vi "RemoteLoader.vi"() -> ()   [LabVIEW 2012]
uses:
  RemoteControl_class/RemoteControl.lvclass
  Light_class/Light.lvclass
  GarageDoor_class/GarageDoor.lvclass
  CeilingFan_class/CeilingFan.lvclass
  Command_class/Command.lvclass
  LightOnCommand_class/LightOnCommand.lvclass
  LightOffCommand_class/LightOffCommand.lvclass
  GarageDoorCloseCommand_class/GarageDoorCloseCommand.lvclass
  GarageDoorOpenCommand_class/GarageDoorOpenCommand.lvclass
  CeilingFanHighCommand_class/CeilingFanHighCommand.lvclass
  CeilingFanLowCommand_class/CeilingFanLowCommand.lvclass
  <userlib>/_LabVIEWCommon/LcError/LcAbort/LcAbort.lvclass
panel:
  in  "stop":bool
  out "error out":errorcluster
  in  "error in (no error)":errorcluster
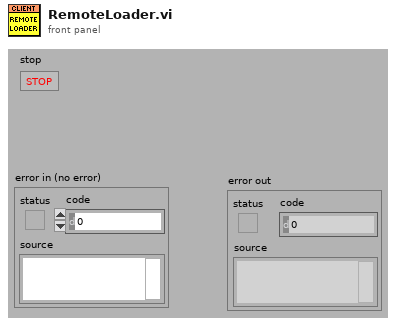
[diagram p1: front panel]
types:
  T1 = cluster{"Remote":refnum<class "RemoteControl.lvclass">, "Light":refnum<class "Light.lvclass">, "GarageDoor":refnum<class "GarageDoor.lvclass">, "CeilingFan":refnum<class "CeilingFan.lvclass">}
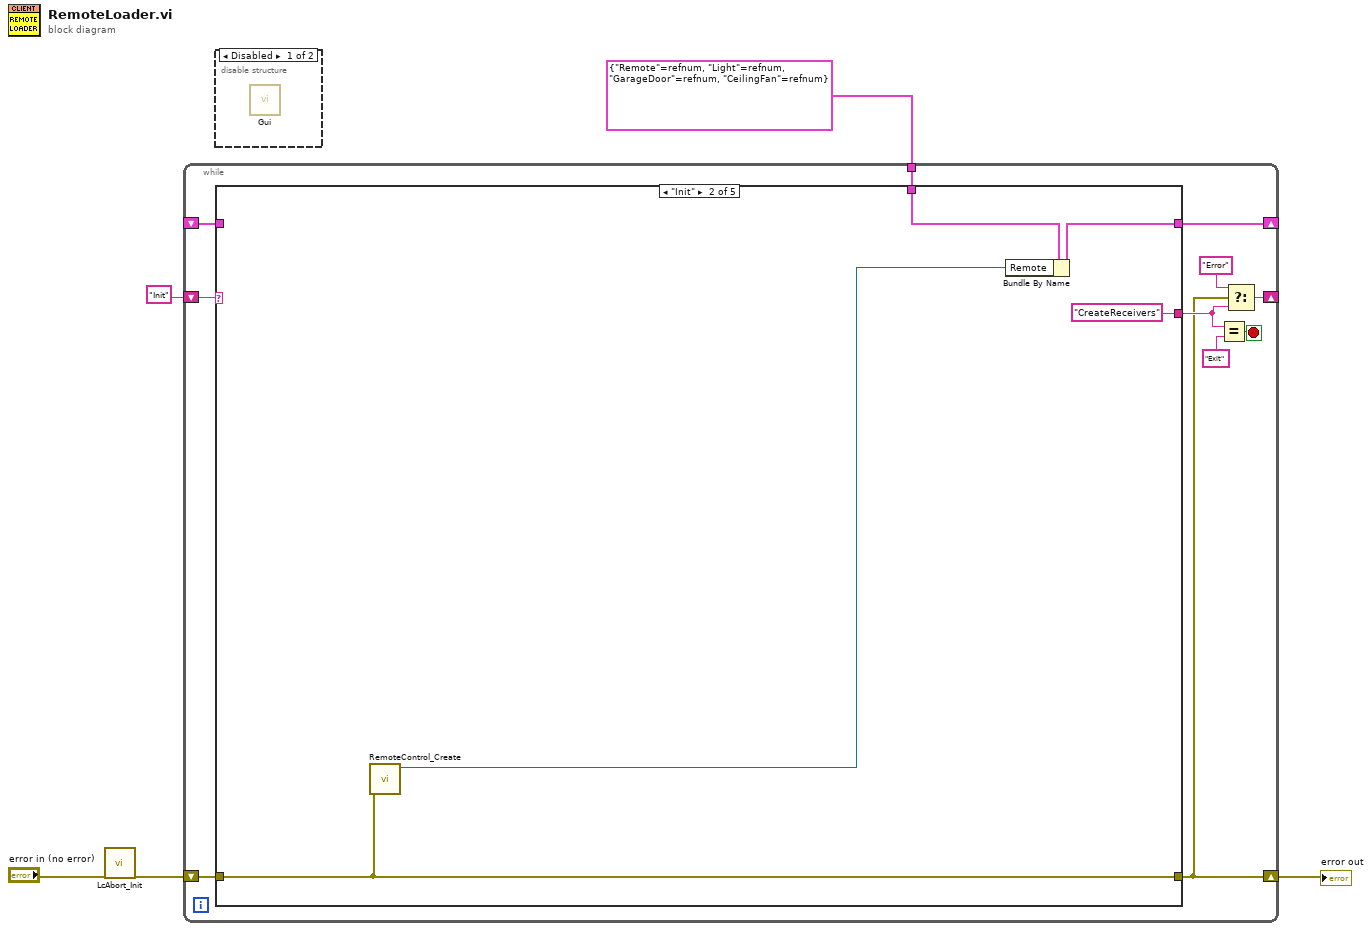
[diagram p0: block diagram]
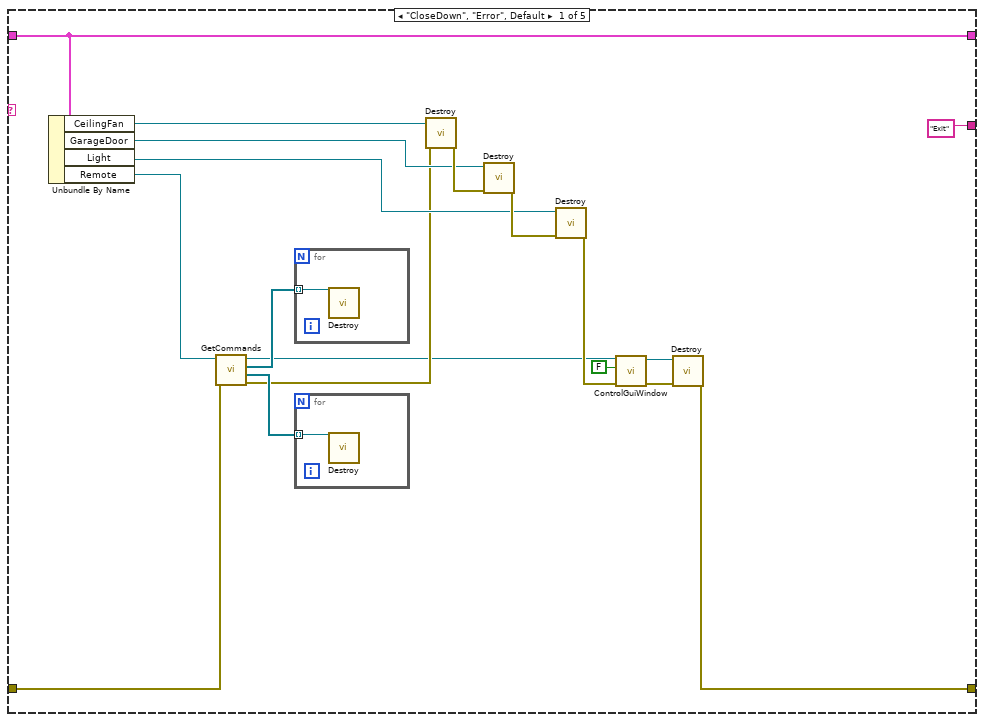
[diagram p3: hidden frame]
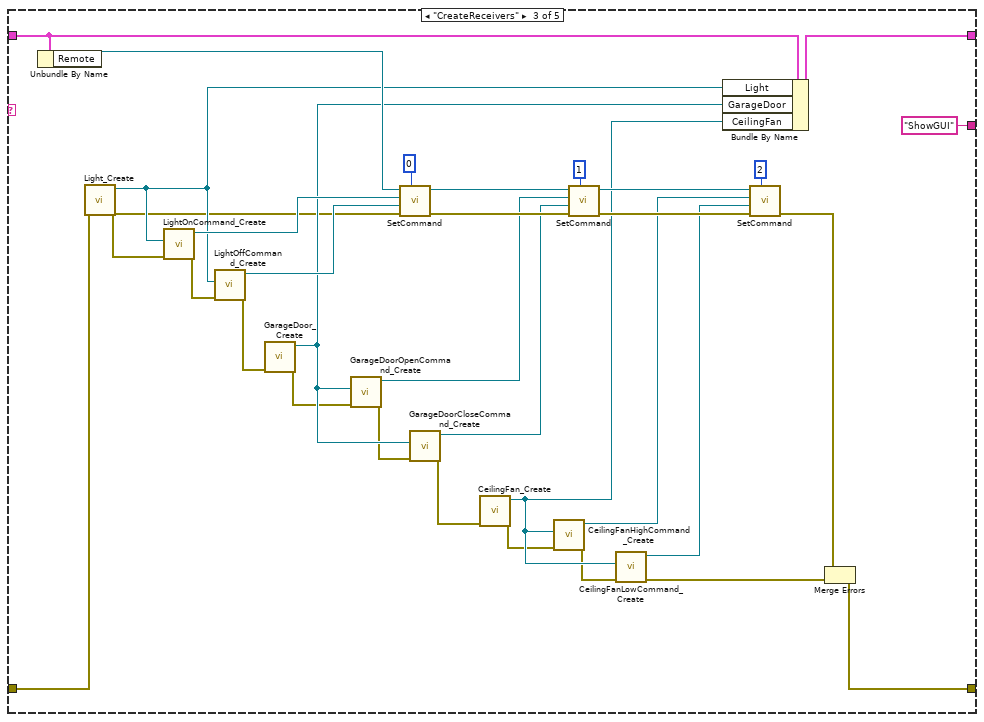
[diagram p4: hidden frame]
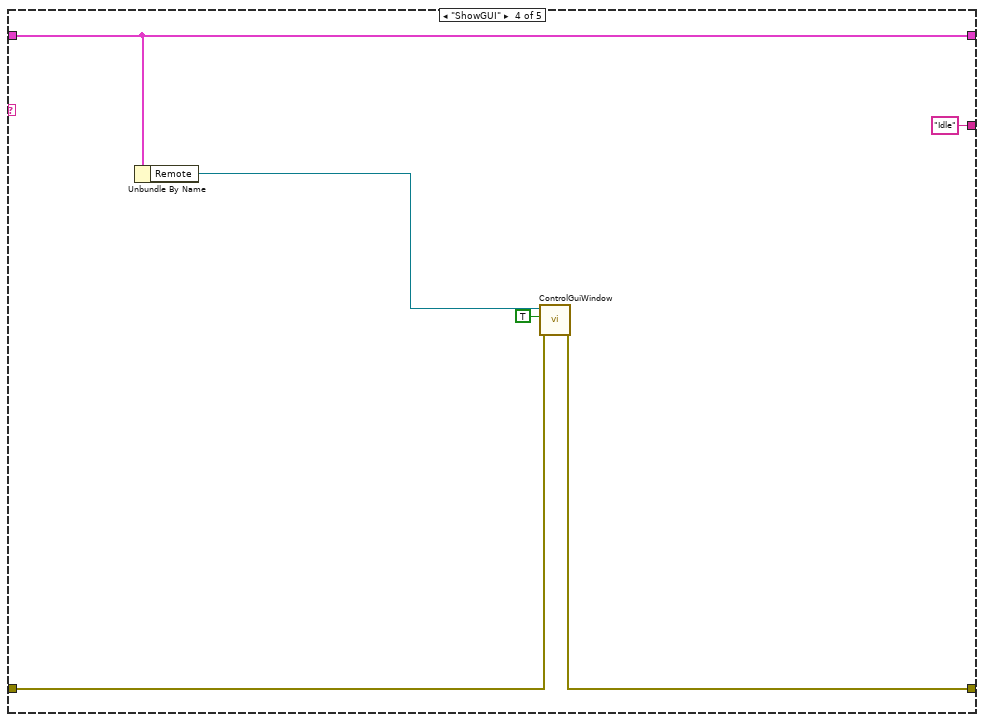
[diagram p5: hidden frame]
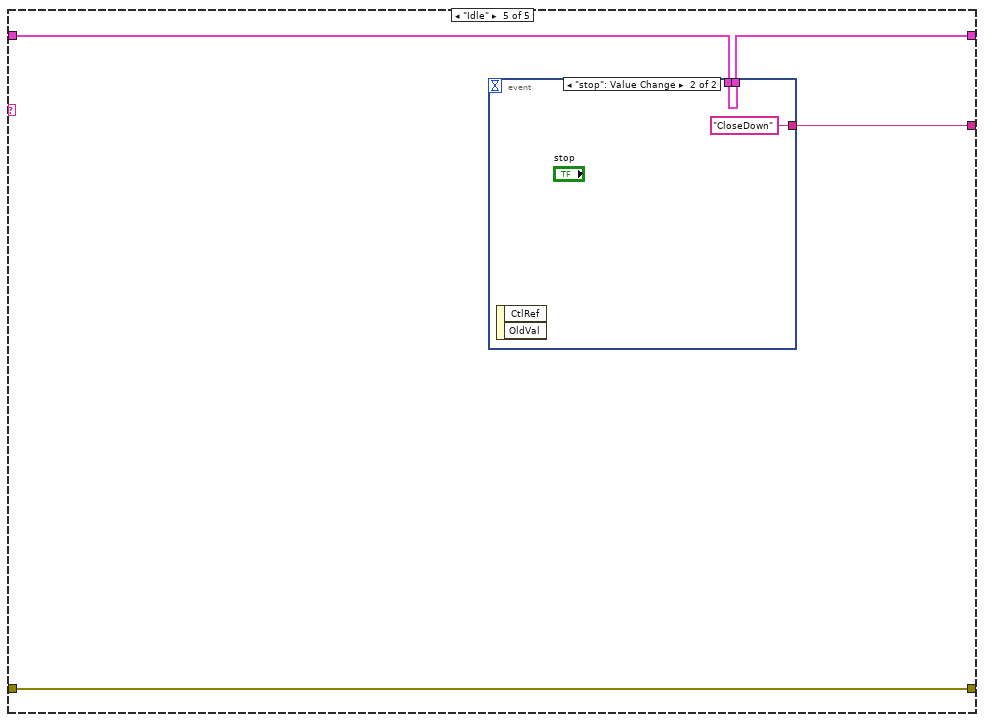
[diagram p6: hidden frame]
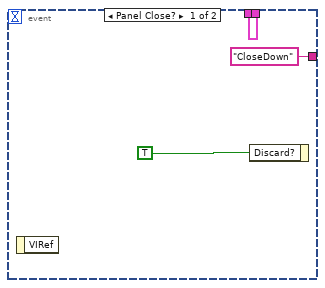
[diagram p7: hidden frame]
diagram:
  n1 = call <userlib>:"LcAbort_Init.vi"("error in (no error)"="error in (no error)") -> ("error out"=w1:errorcluster)  [unwired: 18 in]
  n2 = while {
    shift-right: [w9] -> w4
    shift-left: w1 -> [w16]
    shift-right: [w14] -> _
    shift-left: "Init" -> [w15]
    shift-right: [w8] -> _
    shift-left: _ -> [w7]
    tunnel: T1 {"Remote"=refnum, "Light"=refnum, "GarageDoor"=refnum, "CeilingFan"=refnum} -> [w6]
    stop <- w13 stop-if-true
    n3 = case shown="\"Init\"" w15 {
      tunnel: w16 -> [w19 w39 w57 w79 w80]
      tunnel: [w18 w39 w49 w76 w80] -> w9
      tunnel: ["Exit" "CreateReceivers" "ShowGUI" "Idle" w81] -> w10
      tunnel: [w33 w40 w47 w74 w82] -> w8
      tunnel: w7 -> [w33 _ w48 w74 w83]
      tunnel: w6 -> [_ w37 _ _ _]
      frame "CloseDown", "Error", Default {
        n4 = Unbundle By Name(w33) -> ("CeilingFan"=w32:refnum<class "CeilingFan.lvclass">, "GarageDoor"=w30:refnum<class "GarageDoor.lvclass">, "Light"=w28:refnum<class "Light.lvclass">, "Remote"=w17:refnum<class "RemoteControl.lvclass">)
        n5 = call-dynamic "GetCommands.vi"("error in (no error)"=w19, "reference in"=w17) -> ("error out"=w22:errorcluster, "OfCommands"=w23:refnum<class "Command.lvclass">[], "OnCommands"=w24:refnum<class "Command.lvclass">[], "reference out"=w21:refnum<class "RemoteControl.lvclass">)  [unwired: 6 in]
        n6 = for {
          tunnel: w24 -> [w36] mode=indexing
          n7 = call-dynamic "Destroy.vi"("reference in"=w36) -> ()  [unwired: 9 in, 2 out]
        }
        n8 = for {
          tunnel: w23 -> [w35] mode=indexing
          n9 = call-dynamic "Destroy.vi"("reference in"=w35) -> ()  [unwired: 9 in, 2 out]
        }
        n10 = call-dynamic "Destroy.vi"("error in (no error)"=w22, "reference in"=w32) -> ("error out"=w31:errorcluster)  [unwired: 8 in, 1 out]
        n11 = call-dynamic "Destroy.vi"("error in (no error)"=w31, "reference in"=w30) -> ("error out"=w29:errorcluster)  [unwired: 8 in, 1 out]
        n12 = call-dynamic "Destroy.vi"("error in (no error)"=w29, "reference in"=w28) -> ("error out"=w25:errorcluster)  [unwired: 8 in, 1 out]
        n13 = call "ControlGuiWindow.vi"("error in (no error)"=w25, "ShowProcessWindow"=FALSE, "reference in"=w21) -> ("error out"=w26:errorcluster, "reference out"=w27:refnum<class "RemoteControl.lvclass">)  [unwired: 7 in]
        n14 = call-dynamic "Destroy.vi"("error in (no error)"=w26, "reference in"=w27) -> ("error out"=w18:errorcluster)  [unwired: 8 in, 1 out]
      }
      frame "Init" {
        n15 = call "RemoteControl_Create.vi"("error in (no error)"=w39) -> ("reference out"=w38:refnum<class "RemoteControl.lvclass">)  [unwired: 9 in, 1 out]
        n16 = Bundle By Name(cluster=w37, "Remote"=w38) -> (w40:T1)
      }
      frame "CreateReceivers" {
        n17 = Unbundle By Name(w48) -> ("Remote"=w64:refnum<class "RemoteControl.lvclass">)
        n18 = call "Light_Create.vi"("error in (no error)"=w57) -> ("error out"=w52:errorcluster, "reference out"=w60:refnum<class "Light.lvclass">)  [unwired: 9 in]
        n19 = call "LightOnCommand_Create.vi"("error in (no error)"=w52, "Light"=w60) -> ("error out"=w72:errorcluster, "reference out"=w70:refnum<class "LightOnCommand.lvclass">)  [unwired: 8 in]
        n20 = call "LightOffCommand_Create.vi"("error in (no error)"=w72, "Light"=w60) -> ("error out"=w68:errorcluster, "reference out"=w69:refnum<class "LightOffCommand.lvclass">)  [unwired: 8 in]
        n21 = call "GarageDoor_Create.vi"("error in (no error)"=w68) -> ("error out"=w46:errorcluster, "reference out"=w59:refnum<class "GarageDoor.lvclass">)  [unwired: 9 in]
        n22 = call "GarageDoorOpenCommand_Create.vi"("error in (no error)"=w46, "GarageDoor"=w59) -> ("error out"=w45:errorcluster, "reference out"=w43:refnum<class "GarageDoorOpenCommand.lvclass">)  [unwired: 8 in]
        n23 = call-dynamic "SetCommand.vi"("ButtonIndex(0..n)"=0, "error in (no error)"=w52, "OffCommand"=w69, "OnCommand"=w70, "reference in"=w64) -> ("error out"=w65:errorcluster, "reference out"=w63:refnum<class "RemoteControl.lvclass">)  [unwired: 5 in]
        n24 = call "GarageDoorCloseCommand_Create.vi"("error in (no error)"=w45, "GarageDoor"=w59) -> ("error out"=w44:errorcluster, "reference out"=w42:refnum<class "GarageDoorCloseCommand.lvclass">)  [unwired: 8 in]
        n25 = call "CeilingFan_Create.vi"("error in (no error)"=w44) -> ("error out"=w56:errorcluster, "reference out"=w58:refnum<class "CeilingFan.lvclass">)  [unwired: 9 in]
        n26 = call "CeilingFanHighCommand_Create.vi"("error in (no error)"=w56, "CeilingFan"=w58) -> ("error out"=w55:errorcluster, "reference out"=w54:refnum<class "CeilingFanHighCommand.lvclass">)  [unwired: 8 in]
        n27 = call-dynamic "SetCommand.vi"("ButtonIndex(0..n)"=1, "error in (no error)"=w65, "OffCommand"=w42, "OnCommand"=w43, "reference in"=w63) -> ("error out"=w61:errorcluster, "reference out"=w62:refnum<class "RemoteControl.lvclass">)  [unwired: 5 in]
        n28 = call "CeilingFanLowCommand_Create.vi"("error in (no error)"=w55, "CeilingFan"=w58) -> ("error out"=w51:errorcluster, "reference out"=w53:refnum<class "CeilingFanLowCommand.lvclass">)  [unwired: 8 in]
        n29 = Bundle By Name(cluster=w48, "Light"=w60, "GarageDoor"=w59, "CeilingFan"=w58) -> (w47:T1)
        n30 = call-dynamic "SetCommand.vi"("ButtonIndex(0..n)"=2, "error in (no error)"=w61, "OffCommand"=w53, "OnCommand"=w54, "reference in"=w62) -> ("error out"=w50:errorcluster)  [unwired: 5 in, 1 out]
        n31 = Merge Errors(w50, w51) -> (w49:errorcluster)
      }
      frame "ShowGUI" {
        n32 = Unbundle By Name(w74) -> ("Remote"=w78:refnum<class "RemoteControl.lvclass">)
        n33 = call "ControlGuiWindow.vi"("error in (no error)"=w79, "ShowProcessWindow"=TRUE, "reference in"=w78) -> ("error out"=w76:errorcluster)  [unwired: 7 in, 1 out]
      }
      frame "Idle" {
        n34 = event shown="[1] \"stop\": Value Change" {
          selector: _ -> [_ _]
          dyn-events: _ -> [_ _]
          timeout: _ -> [_ _]
          tunnel: w83 -> [w84 w87]
          tunnel: [w84 w87] -> w82
          tunnel: ["CloseDown" "CloseDown"] -> w81
          event Panel Close? {
            n35 = event-data() -> ()  [unwired: 1 in, 1 out]
            n36 = event-data("Discard?"=TRUE) -> ()  [unwired: 1 in, 1 out]
          }
          event "stop": Value Change {
            n37 = event-data() -> ()  [unwired: 1 in, 2 out]
          }
        }
      }
    }
    n38 = Equal?(x=w10, y="Exit") -> (x = y?=w13:bool)
    n39 = Select(t="Error", s=w9, f=w10) -> (s? t:f=w14:string)
  }
  "error out" <- w4
  n40 = disable-structure shown="Disabled" {
    frame Disabled {
      n41 = call "Gui.vi"() -> ()  [unwired: 18 in, 2 out]
    }
    frame Enabled {
    }
  }
